vi "tvac_gui_v3.vi"() -> ()   [LabVIEW 2016]
uses:
  <vilib>/httpClient/LabVIEWHTTPClient.lvlib
  <vilib>/httpClient/ClientHandle.ctl
  msg7171_linux.llb/send single message.vi
  <vilib>/httpClient/POSTBuffer.vi
panel:
  in  "alarm":i32
  in  "NumberTCs":i32=10
  in  "Tab Control":enum32{"Page 1", "Page 2"}(tab)
  in  "Zone 1":T1 {"Ring" items=["Average", "Maximum", "Minimum", ""]}
  in  "Graphing Selection":u16(ring) items=["User Selection", "Graph All Thermocouples", "Clear Graph"]
  in  "Time Scale":u16(ring) items=["Minutes", "Hours", "Seconds"]
  out "Waveform Chart":waveform(dbl)[](graph)
  out "Thermocouples":T2(array[cluster])
  in  "exit":bool
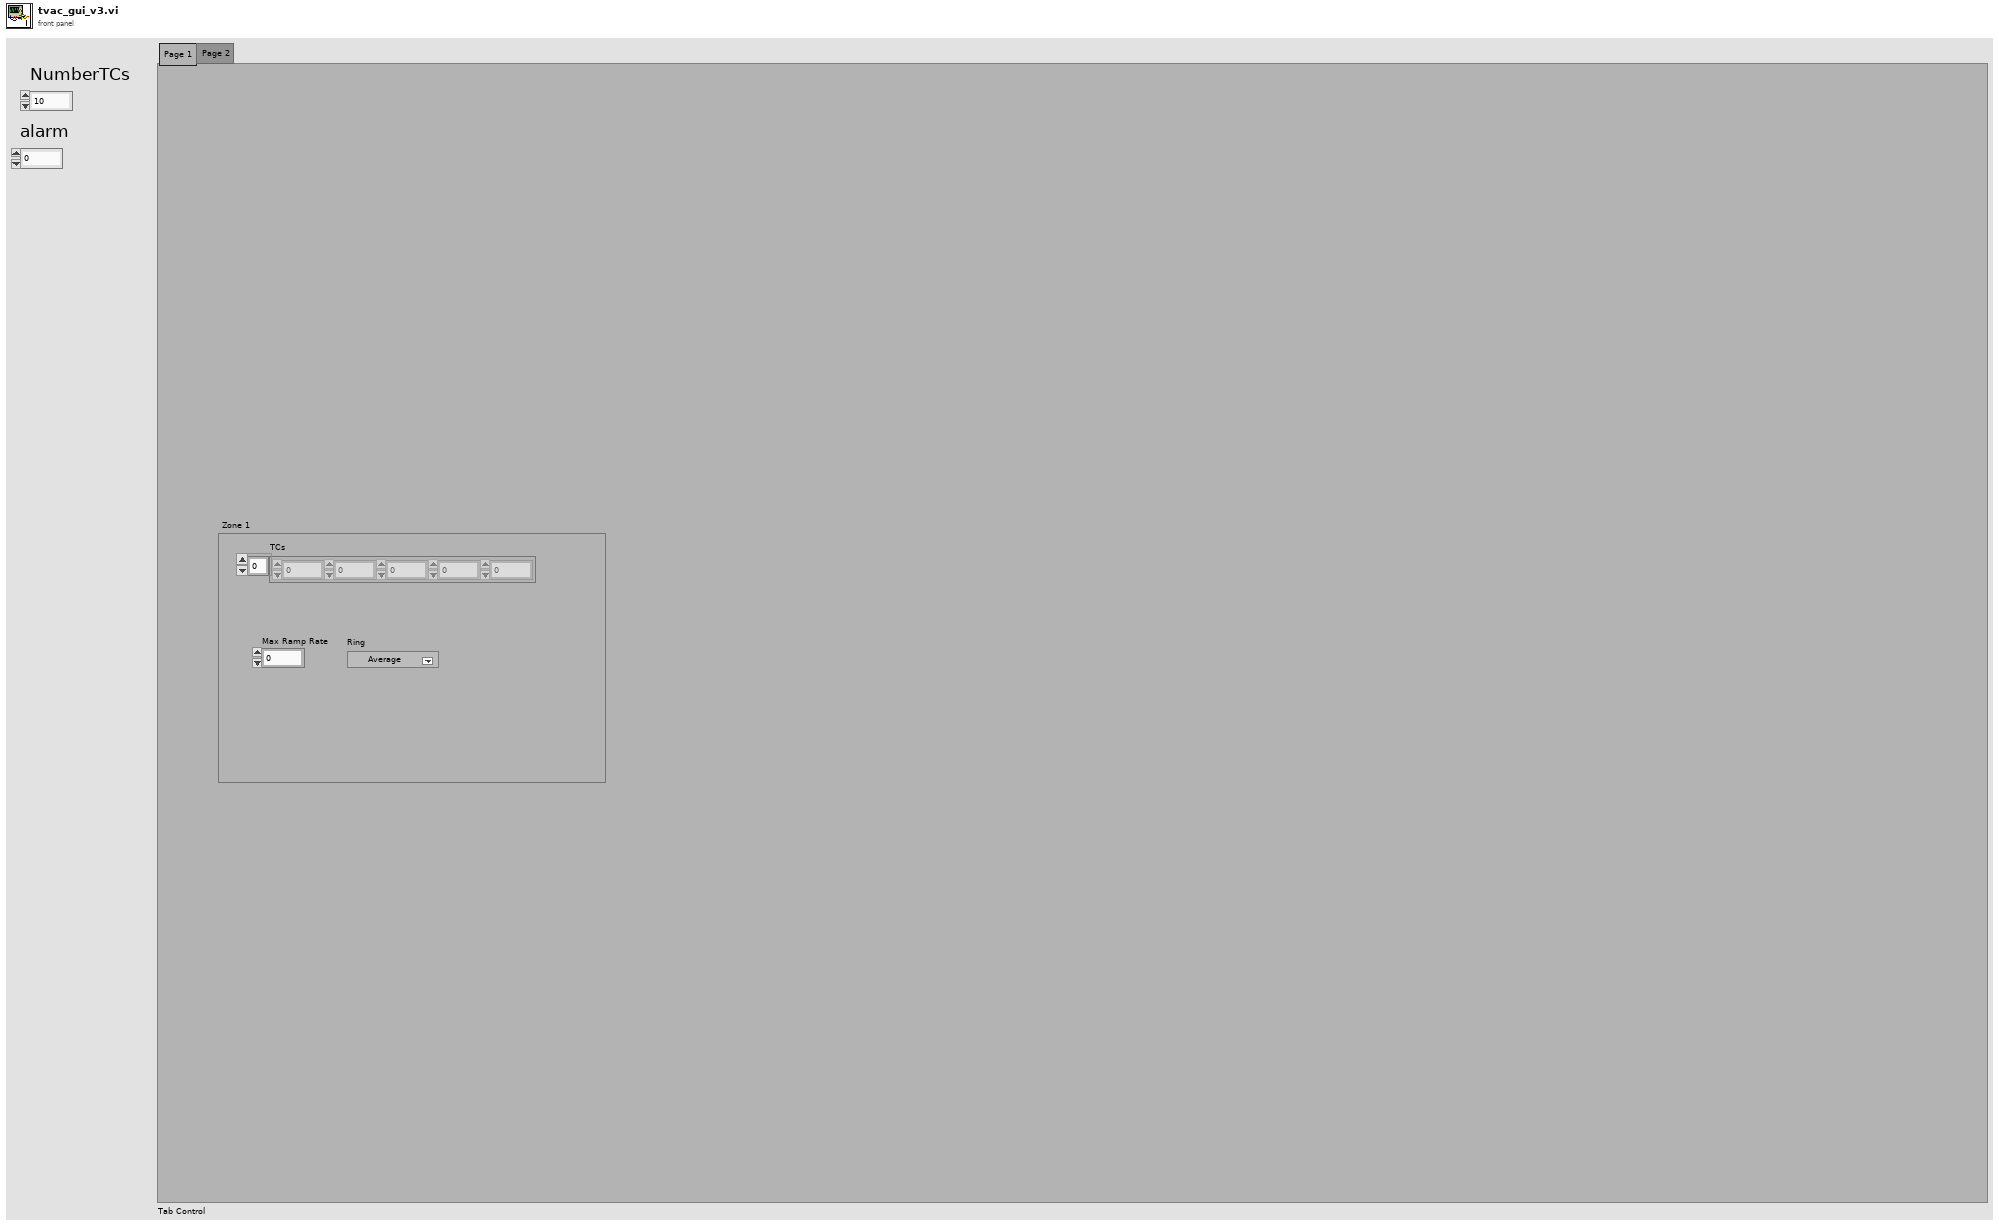
[diagram p1: front panel]
types:
  T1 = cluster{"Ring":u16, "Max Ramp Rate":dbl, "TCs":dbl[]}
  T2 = cluster{"TC Label":string, "Alarm Status":string, "Alarm Color":u32, "Temperature":string, "PlotColor":u32, "Graph On/Off":u32}[][]
  T3 = typedef "LabVIEWHTTPClient.lvlib/ClientHandle.ctl" = refnum<k1>
  T4 = cluster{"go":bool, "Http session":T3, "URL prefex":string}
  T5 = typedef "LVPoint32TypeDef.ctl" = cluster{"Horizontal":i32, "Vertical":i32}
  T6 = typedef "LVPositionTypeDef.ctl" = cluster{"Left":i32, "Top":i32}
  T7 = cluster{"TC Label":string, "Alarm Status":string, "Alarm Color":u32, "Temperature":string, "PlotColor":u32, "Graph On/Off":u32}
  T8 = typedef "LVRangeTypeDef.ctl" = cluster{"Minimum":dbl, "Maximum":dbl, "Increment":dbl, "Minor Increment":dbl, "Start":dbl}
  T9 = cluster{"time":string, "tcs":cluster{"thermocouple":i32, "time":i32, "temp":i32, "working":i32, "alarm":i32}[]}
  T10 = cluster{"thermocouple":i32, "time":i32, "temp":i32, "working":i32, "alarm":i32}[]
  T11 = cluster{"thermocouple":i32, "time":i32, "temp":i32, "working":i32, "alarm":i32}
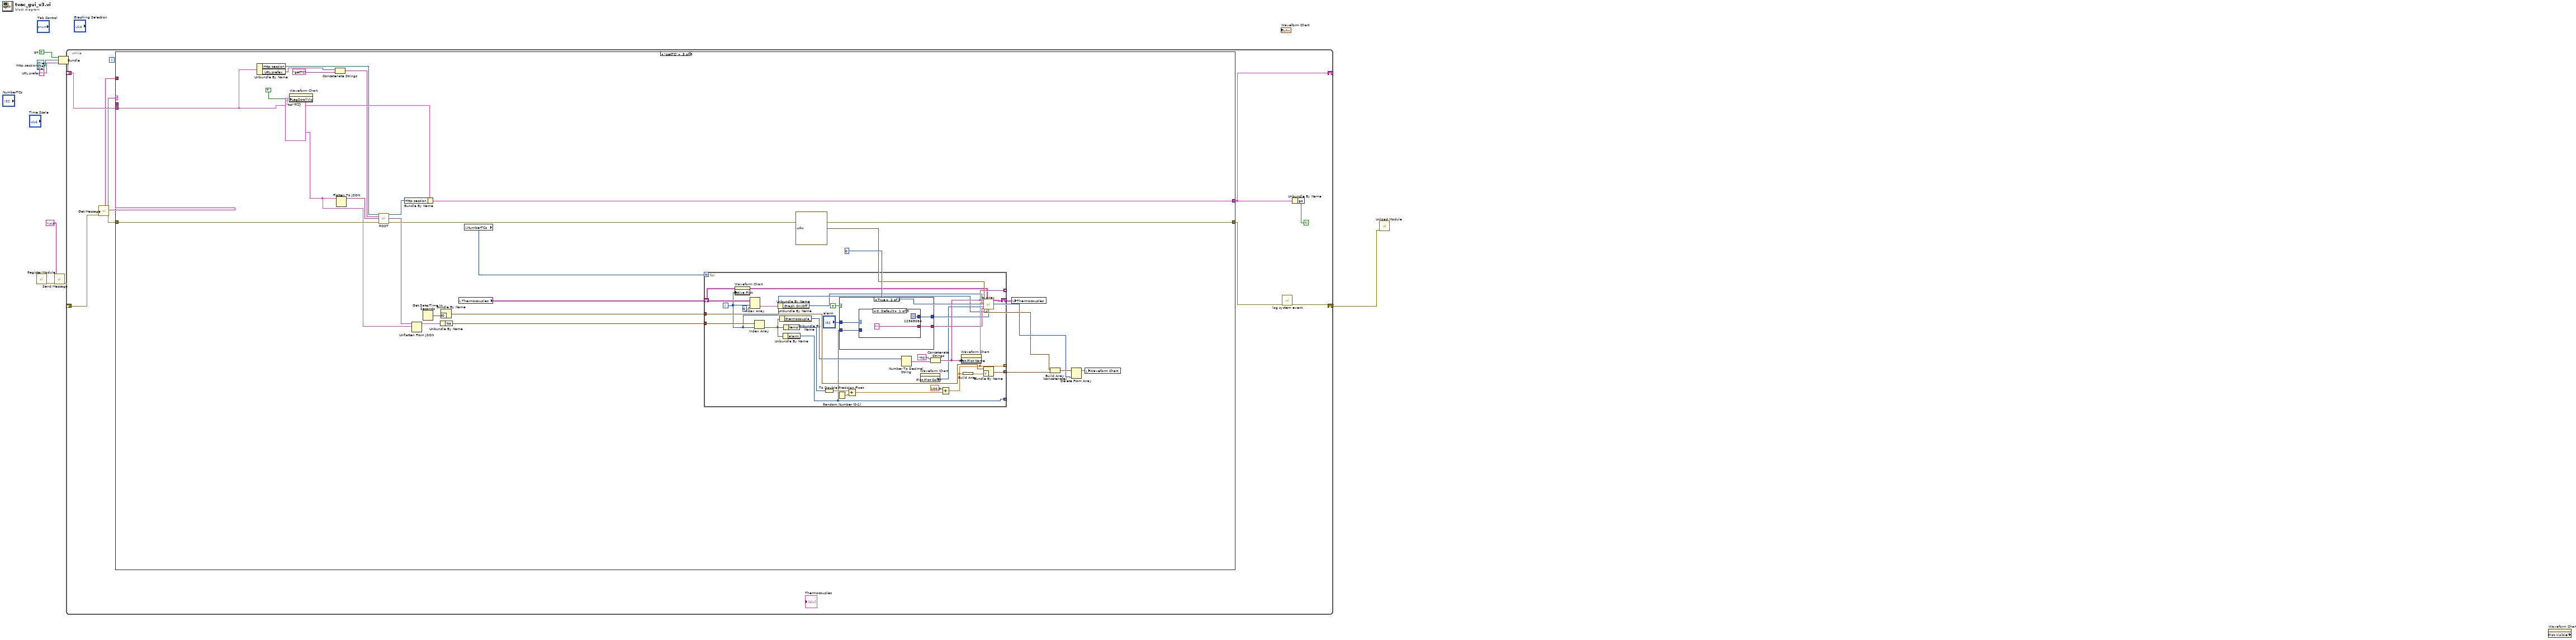
[diagram p0: block diagram]
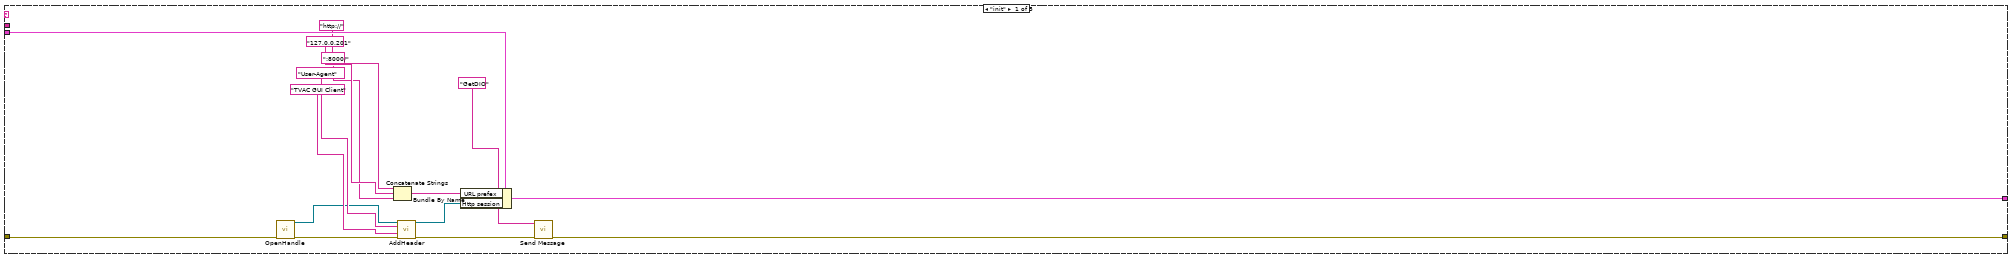
[diagram p2: hidden frame]
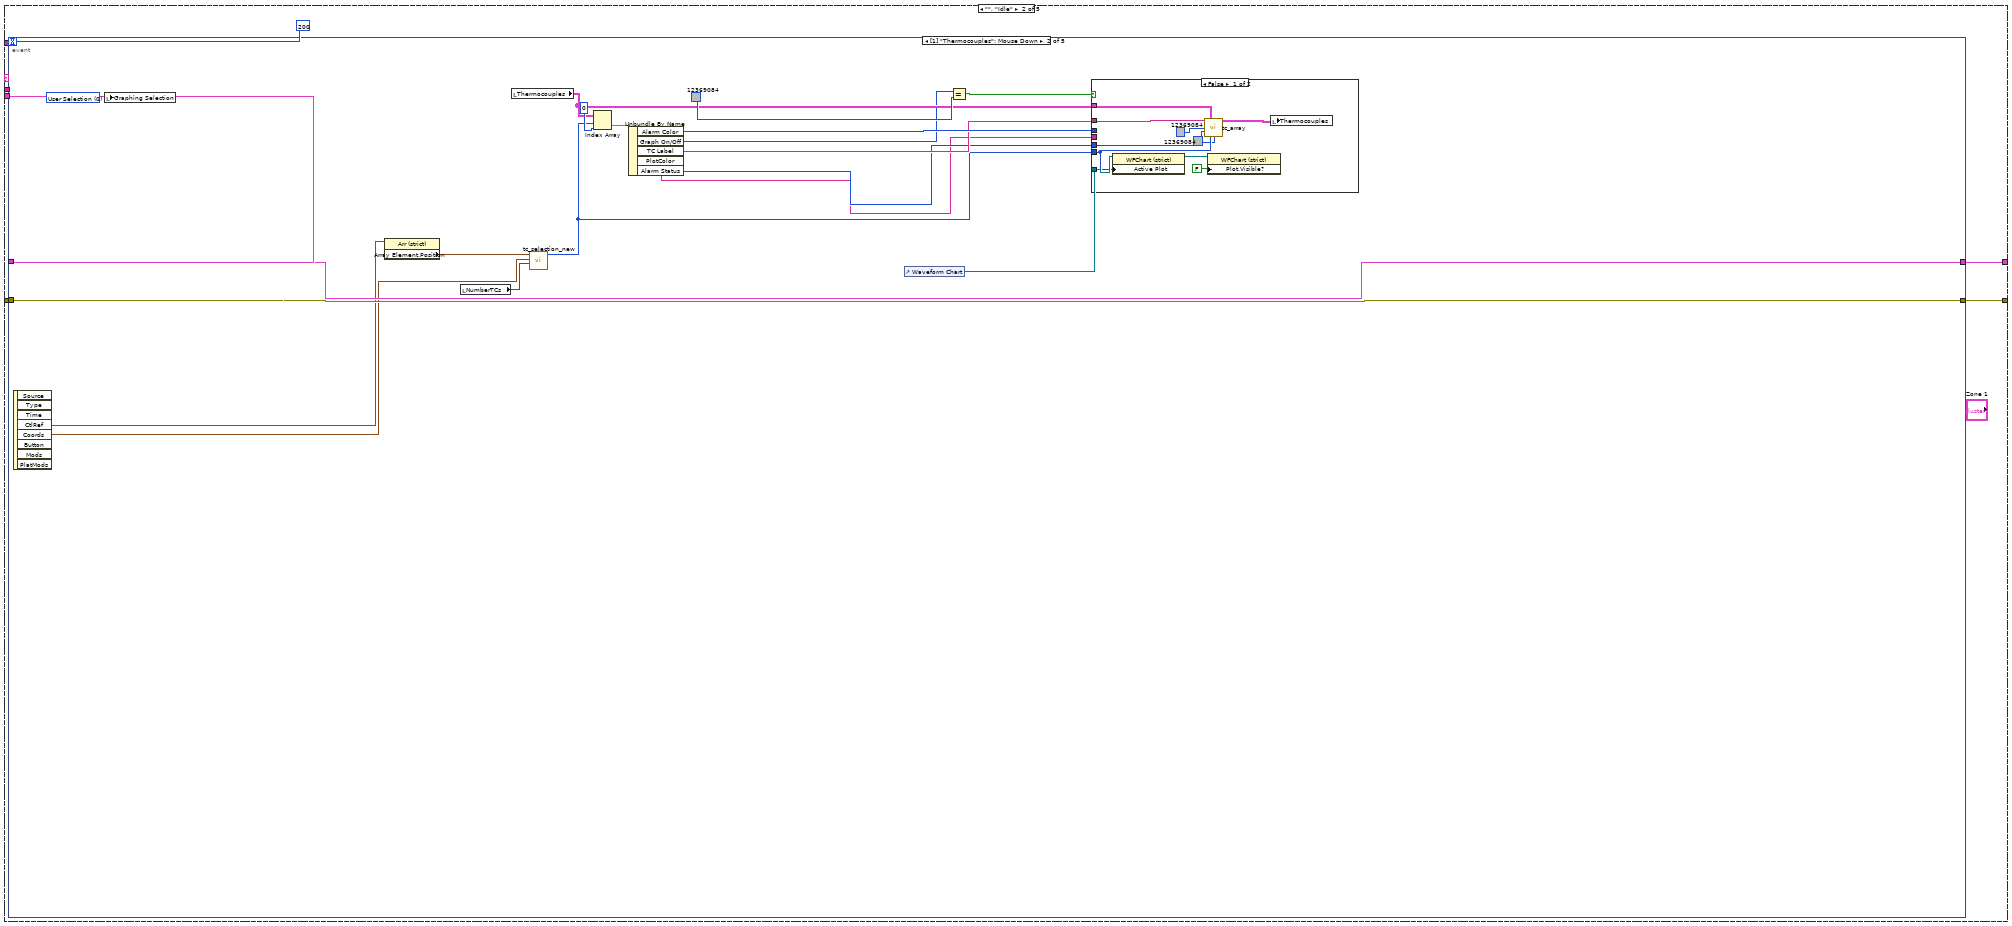
[diagram p3: hidden frame]
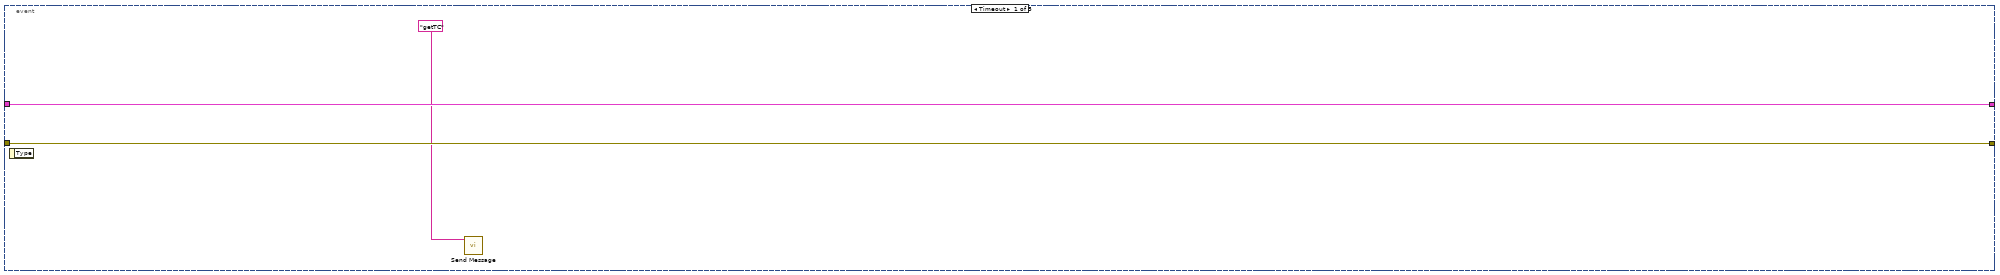
[diagram p4: hidden frame]
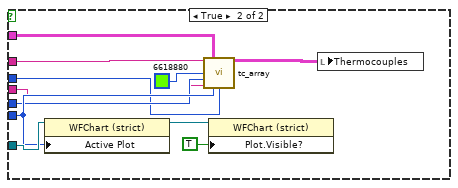
[diagram p5: hidden frame]
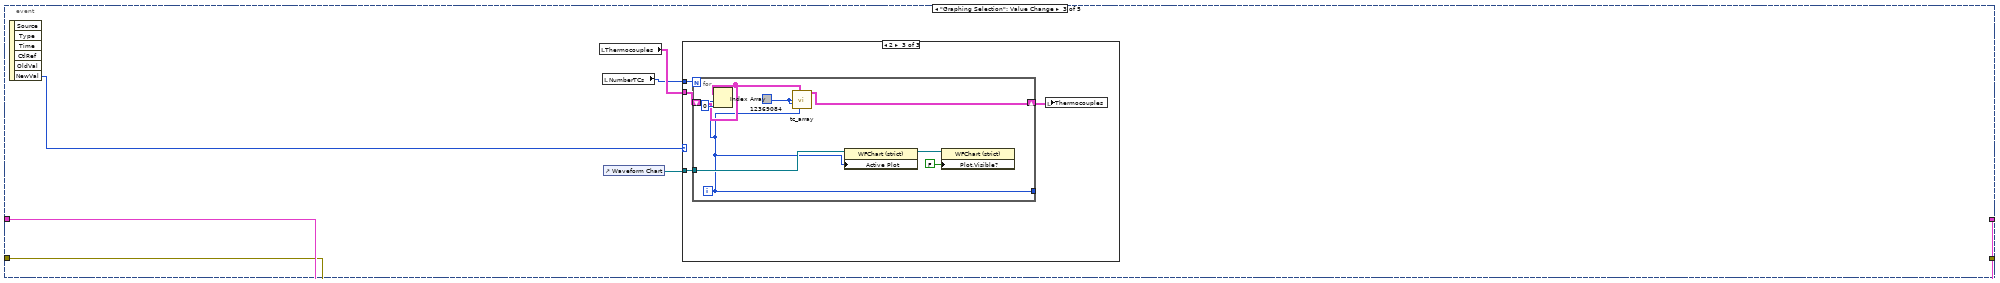
[diagram p6: hidden frame]
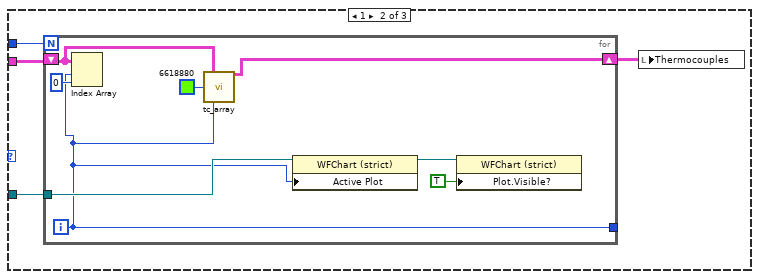
[diagram p8: hidden frame]
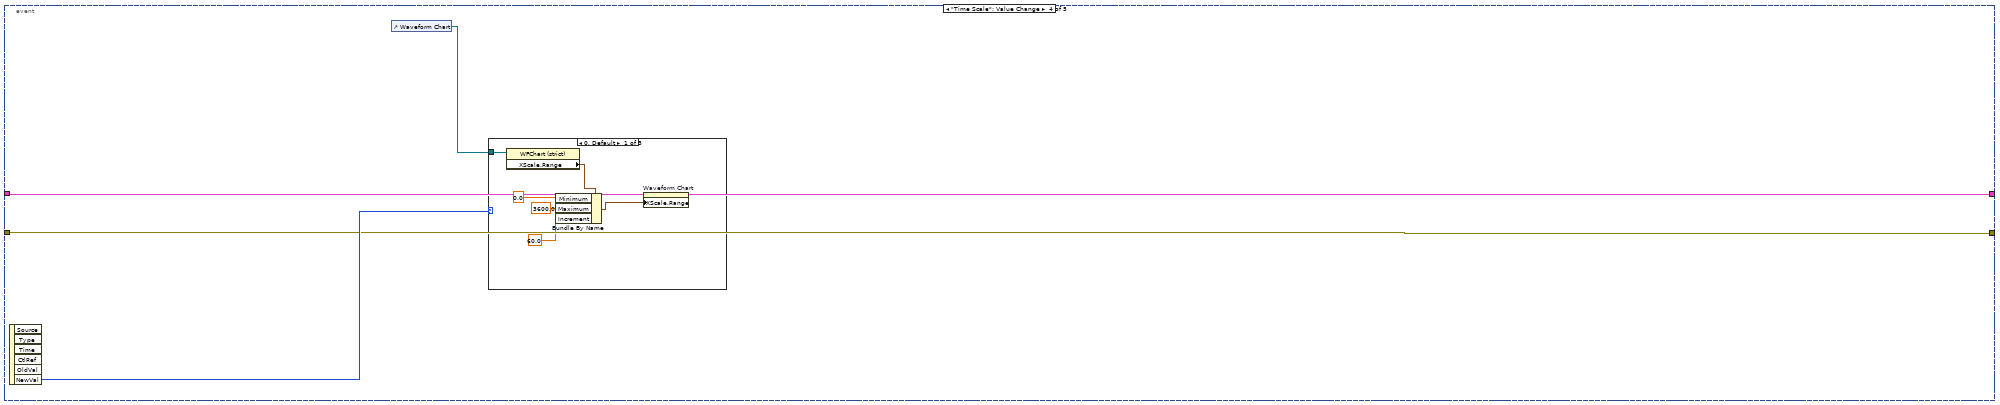
[diagram p9: hidden frame]
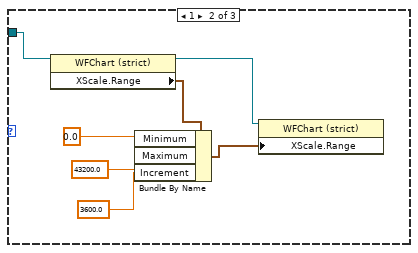
[diagram p10: hidden frame]
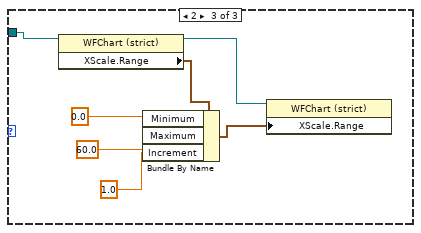
[diagram p11: hidden frame]
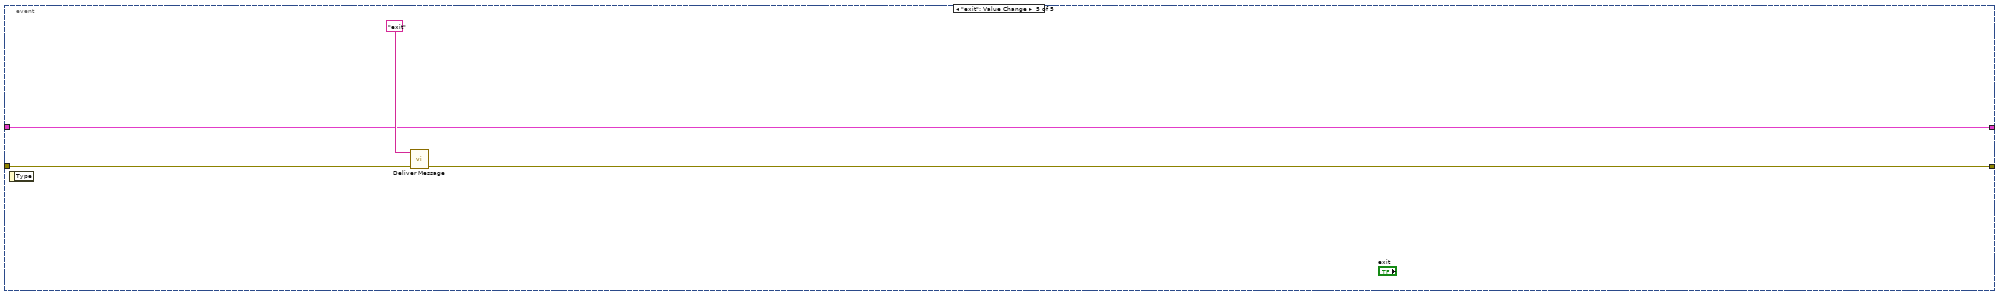
[diagram p12: hidden frame]
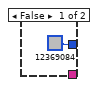
[diagram p13: hidden frame]
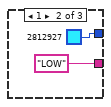
[diagram p14: hidden frame]
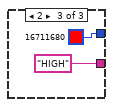
[diagram p15: hidden frame]
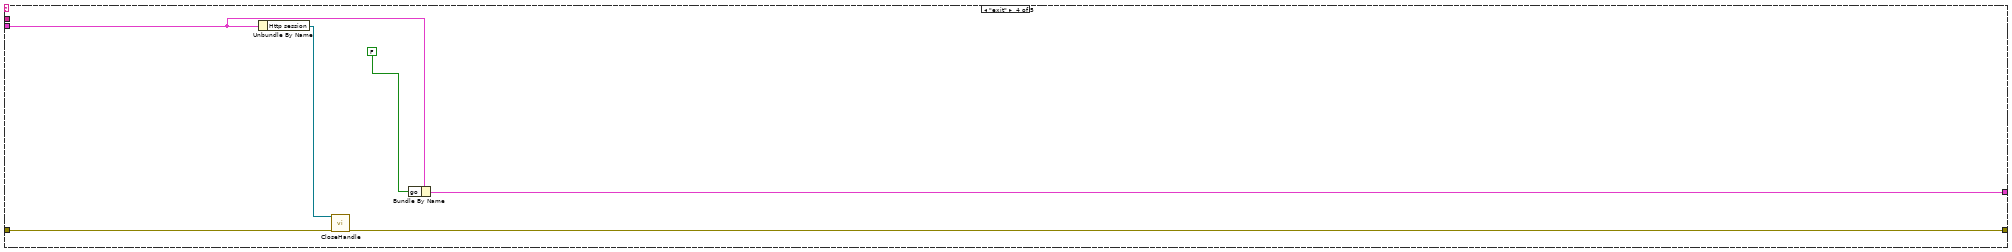
[diagram p16: hidden frame]
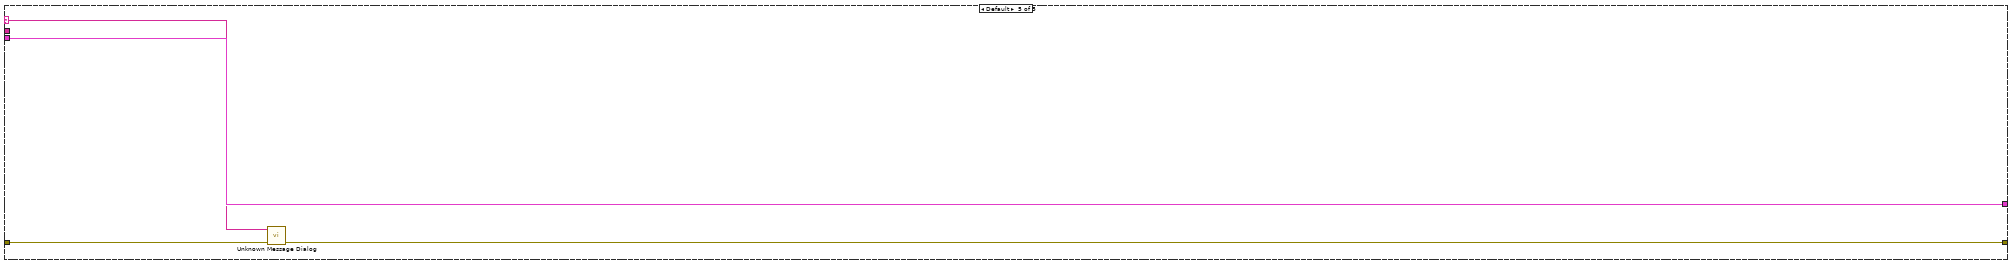
[diagram p17: hidden frame]
diagram:
  w4 = ""  # URL prefex
  w5 = T3 refnum  # Http session
  w6 = TRUE  # go
  n1 = call "Register Module.vi"() -> ("error out"=w2:errorcluster)  [unwired: 10 in, 1 out]
  n2 = call-poly "Send Message.vi"("error in (no error)"=w2, "event"="init") -> ("error out"=w1:errorcluster)  [unwired: 9 in]
  n3 = Bundle("go"=w6, "Http session"=w5, "URL prefex"=w4) -> (w8:T4)  [unwired: 1 in]
  n4 = while {
    shift-left: w8 -> [w15]
    shift-right: [w13] -> _
    shift-right: [w12] -> w7
    shift-left: w1 -> [w18]
    stop <- w9 continue-if-true
    n5 = call "Get Message.vi"("error in (no error)"=w18) -> ("error out"=w16:errorcluster, "event buffer"=w17:string, "event"=w14:string, "source"=w10:string)  [unwired: 7 in]
    n6 = case shown="\"getTC\"" w14 {
      selector: w14 -> [_ _ _ _ w210]
      tunnel: [w24 w35 w162 w208 w212] -> w13
      tunnel: w15 -> [w33 w34 w160 w203 w212]
      tunnel: w17 -> [_ _ _ _ _]
      tunnel: w16 -> [w28 w36 w164 w206 w211]
      tunnel: [w20 w38 w163 w205 w209] -> w11
      tunnel: w10 -> [_ _ _ _ _]
      frame "init" {
        n7 = call <vilib>:"OpenHandle.vi"("error in (no error)"=w28) -> ("client handle out"=w29:T3, "error out"=w32:errorcluster)  [unwired: 13 in]
        n8 = Concatenate Strings("http://" ("url"), "127.0.0.201" ("Address"), ":8000/" ("url")) -> (w23:string)
        n9 = call <vilib>:"AddHeader.vi"("client handle"=w29, "header"="User-Agent", "value"="TVAC GUI Client", "error in (no error)"=w32) -> ("client handle out"=w22:T3, "error out"=w21:errorcluster)  [unwired: 10 in]
        n10 = Bundle By Name(cluster=w33, "URL prefex"=w23, "Http session"=w22) -> (w24:T4)
        n11 = call-poly "Send Message.vi"("error in (no error)"=w21, "event"="GetDIO") -> ("error out"=w20:errorcluster)  [unwired: 9 in]
      }
      frame "", "Idle" {
        n12 = event shown="[1] \"Thermocouples\": Mouse Down" {
          selector: _ -> [_ _ _ _ _]
          dyn-events: _ -> [_ _ _ _ _]
          timeout: 200 ("milliseconds to wait") -> [_ _ _ _ _]
          tunnel: w36 -> [w40 w60 w86 w113 w139]
          tunnel: [w40 w60 w86 w113 w138] -> w38
          tunnel: [w41 w59 w87 w114 w136] -> w35
          tunnel: w34 -> [w41 w59 w87 w114 w136]
          event Timeout {
            n13 = event-data() -> ()  [unwired: 1 in, 1 out]
            n14 = call-poly "Send Message.vi"("event"="getTC") -> ()  [unwired: 10 in, 1 out]
          }
          event "Thermocouples": Mouse Down {
            w42 = u16 0 items=["User Selection", "Graph All Thermocouples", "Clear Graph"] ("Graphing Selection")
            n15 = event-data() -> ("CtlRef"=w56:refnum<vi>, "Coords"=w57:T5)  [unwired: 1 in, 6 out]
            n16 = local write "Graphing Selection"(w42) -> ()
            n17 = property class="Arr (strict)"(reference=w56) -> ("Array Element.Position"=w58:T6)  [unwired: 1 in, 2 out]
            n18 = local read "NumberTCs"() -> (w48:i32)
            n19 = local read "Thermocouples"() -> (w50:T2)
            n20 = call "tc_selection_new.vi"("Numeric 2"=w48, "Coords"=w57, "Position"=w58) -> ("Numeric"=w44:i32)  [unwired: 8 in]
            n21 = Index Array(array=w50, index (row)=w44, index (col)=0 ("disabled index (col)")) -> (element=w53:T7)
            n22 = Unbundle By Name(w53) -> ("Alarm Color"=w49:u32, "Graph On/Off"=w47:u32, "TC Label"=w46:string, "PlotColor"=w45:u32, "Alarm Status"=w43:string)
            n23 = control-ref of="Waveform Chart"() -> (w51:refnum<vi>)
            n24 = Equal?(x=w47, y=u32 12369084) -> (x = y?=w52:bool)
            n25 = case shown="False" w52 {
              tunnel: w44 -> [w62 w74]
              tunnel: w51 -> [w68 w79]
              tunnel: w50 -> [w64 w76]
              tunnel: w49 -> [_ w72]
              tunnel: w46 -> [w66 w78]
              tunnel: w45 -> [w63 w73]
              tunnel: w43 -> [_ w71]
              frame False {
                n26 = property on="Property Node" class="WFChart (strict)"(reference=w68, "Active Plot"=w62) -> (reference out=w69:refnum<vi>)  [unwired: 1 in, 1 out]
                n27 = call "tc_array.vi"("TC Label"=w66, "output array 2"=w64, "Graph ON/OFF"=u32 12369084, "Plot Color"=w63, "index (row)"=w62, "AlarmColor"=u32 12369084) -> ("output array"=w65:T2)  [unwired: 9 in]
                n28 = property class="WFChart (strict)"(reference=w69, "Plot.Visible?"=FALSE ("Plot.Visible")) -> ()  [unwired: 1 in, 2 out]
                n29 = local write "Thermocouples"(w65) -> ()
              }
              frame True {
                n30 = property class="WFChart (strict)"(reference=w79, "Active Plot"=w74) -> (reference out=w80:refnum<vi>)  [unwired: 1 in, 1 out]
                n31 = call "tc_array.vi"("TC Label"=w78, "output array 2"=w76, "Graph ON/OFF"=u32 6618880, "Plot Color"=w73, "Alarm String"=w71, "index (row)"=w74, "AlarmColor"=w72) -> ("output array"=w75:T2)  [unwired: 8 in]
                n32 = property class="WFChart (strict)"(reference=w80, "Plot.Visible?"=TRUE ("Plot.Visible")) -> ()  [unwired: 1 in, 2 out]
                n33 = local write "Thermocouples"(w75) -> ()
              }
            }
          }
          event "Graphing Selection": Value Change {
            n34 = event-data() -> ("NewVal"=w82:u16)  [unwired: 1 in, 5 out]
            n35 = local read "Thermocouples"() -> (w85:T2)
            n36 = local read "NumberTCs"() -> (w83:i32)
            n37 = control-ref of="Waveform Chart"() -> (w84:refnum<vi>)
            n38 = case shown="2" w82 {
              tunnel: w85 -> [_ w91 w102]
              tunnel: w84 -> [_ w90 w101]
              tunnel: w83 -> [_ w89 w103]
              frame 0, Default {
              }
              frame 1 {
                n39 = for {
                  N: w89 -> [_]
                  tunnel: w90 -> [w96]
                  tunnel: [w95] -> _
                  shift-right: [w93] -> w88
                  shift-left: w91 -> [w94]
                  i -> [w95]
                  n40 = Index Array(array=w94, index (row)=w95, index (col)=0 ("disabled index (col)")) -> ()  [unwired: 1 out]
                  n41 = call "tc_array.vi"("output array 2"=w94, "Graph ON/OFF"=u32 6618880, "index (row)"=w95) -> ("output array"=w93:T2)  [unwired: 12 in]
                  n42 = property class="WFChart (strict)"(reference=w96, "Active Plot"=w95) -> (reference out=w98:refnum<vi>)  [unwired: 1 in, 1 out]
                  n43 = property class="WFChart (strict)"(reference=w98, "Plot.Visible?"=TRUE ("Plot.Visible")) -> ()  [unwired: 1 in, 2 out]
                }
                n44 = local write "Thermocouples"(w88) -> ()
              }
              frame 2 {
                n45 = for {
                  N: w103 -> [_]
                  tunnel: w101 -> [w108]
                  tunnel: [w106] -> _
                  shift-right: [w104] -> w100
                  shift-left: w102 -> [w107]
                  i -> [w106]
                  w105 = u32 12369084
                  n46 = Index Array(array=w107, index (row)=w106, index (col)=0 ("disabled index (col)")) -> ()  [unwired: 1 out]
                  n47 = call "tc_array.vi"("output array 2"=w107, "Graph ON/OFF"=w105, "Plot Color"=w105, "index (row)"=w106) -> ("output array"=w104:T2)  [unwired: 11 in]
                  n48 = property class="WFChart (strict)"(reference=w108, "Active Plot"=w106) -> (reference out=w110:refnum<vi>)  [unwired: 1 in, 1 out]
                  n49 = property class="WFChart (strict)"(reference=w110, "Plot.Visible?"=FALSE ("Plot.Visible")) -> ()  [unwired: 1 in, 2 out]
                }
                n50 = local write "Thermocouples"(w100) -> ()
              }
            }
          }
          event "Time Scale": Value Change {
            n51 = event-data() -> ("NewVal"=w115:u16)  [unwired: 1 in, 5 out]
            n52 = control-ref of="Waveform Chart"() -> (w112:refnum<vi>)
            n53 = case shown="0, Default" w115 {
              tunnel: w112 -> [w119 w123 w130]
              frame 0, Default {
                n54 = property on="Property Node" class="WFChart (strict)"(reference=w119) -> ("XScale.Range"=w121:T8)  [unwired: 1 in, 2 out]
                n55 = Bundle By Name(cluster=w121, "Minimum"=0.0, "Maximum"=3600.0, "Increment"=60.0) -> (w120:T8)
                n56 = property on="Waveform Chart" class="WFChart (strict)"("XScale.Range"=w120) -> ()  [unwired: 2 in, 2 out]
              }
              frame 1 {
                n57 = property on="Property Node" class="WFChart (strict)"(reference=w123) -> (reference out=w122:refnum<vi>, "XScale.Range"=w128:T8)  [unwired: 1 in, 1 out]
                n58 = Bundle By Name(cluster=w128, "Minimum"=0.0, "Maximum"=43200.0, "Increment"=3600.0) -> (w124:T8)
                n59 = property on="Property Node" class="WFChart (strict)"(reference=w122, "XScale.Range"=w124) -> ()  [unwired: 1 in, 2 out]
              }
              frame 2 {
                n60 = property on="Property Node" class="WFChart (strict)"(reference=w130) -> (reference out=w129:refnum<vi>, "XScale.Range"=w135:T8)  [unwired: 1 in, 1 out]
                n61 = Bundle By Name(cluster=w135, "Minimum"=0.0, "Maximum"=60.0, "Increment"=1.0) -> (w131:T8)
                n62 = property on="Property Node" class="WFChart (strict)"(reference=w129, "XScale.Range"=w131) -> ()  [unwired: 1 in, 2 out]
              }
            }
          }
          event "exit": Value Change {
            n63 = event-data() -> ()  [unwired: 1 in, 1 out]
            n64 = call "Deliver Message.vi"("error in (no error)"=w139, "event"="exit") -> ("error out"=w138:errorcluster)  [unwired: 9 in]
          }
        }
      }
      frame "getTC" {
        w153 = T9 {"time"="", "tcs"=[]}
        n65 = Unbundle By Name(w160) -> ("Http session"=w159:T3, "URL prefex"=w157:string)
        n66 = property on="Waveform Chart" class="WFChart (strict)"("LegScrollVis"=TRUE ("Legend:Scrollbar Visible")) -> ()  [unwired: 2 in, 2 out]
        n67 = Concatenate Strings(w157, "getTC" ("url")) -> (w158:string)
        n68 = Flatten To JSON(anything=w153) -> (JSON string=w155:string)  [unwired: 2 in, 1 out]
        n69 = call-poly <vilib>:"POST.vi"("client handle"=w159, "url"=w158, "buffer"=w155, "error in (no error)"=w164) -> ("client handle out"=w161:T3, "body"=w154:string, "error out"=w163:errorcluster)  [unwired: 8 in, 1 out]
        n70 = Bundle By Name(cluster=w160, "Http session"=w161) -> (w162:T4)
        n71 = Unflatten From JSON(JSON string=w154, type and defaults=w153) -> (value=w152:T9)  [unwired: 5 in, 1 out]
        n72 = Get Date/Time In Seconds() -> (seconds since 1Jan1904=w148:timestamp)
        n73 = Unbundle By Name(w152) -> ("tcs"=w151:T10)
        n74 = Bundle By Name("t0"=w148) -> (w147:waveform(dbl))  [unwired: 1 in]
        n75 = local read "Thermocouples"() -> (w143:T2)
        n76 = local read "NumberTCs"() -> (w140:i32)
        n77 = for {
          N: w140 -> [_]
          tunnel: w151 -> [w191]
          tunnel: w147 -> [w189]
          tunnel: [w190] -> w146 mode=indexing
          tunnel: [w172] -> _ mode=indexing
          tunnel: [w171] -> _ mode=indexing
          tunnel: [w174] -> _ mode=indexing
          shift-right: [w173] -> w144
          shift-left: w143 -> [w170]
          i -> [w167]
          n78 = property on="Waveform Chart" class="WFChart (strict)"("Active Plot"=w167) -> ()  [unwired: 2 in, 2 out]
          n79 = Index Array(array=w170, index (row)=w167, index (col)=0 ("disabled index (col)")) -> (element=w177:T7)
          n80 = Index Array(array=w191, index=w167) -> (element=w181:T11)
          n81 = Unbundle By Name(w177) -> ("Graph On/Off"=w165:u32)
          n82 = Unbundle By Name(w181) -> ("thermocouple"=w187:i32)
          n83 = Unbundle By Name(w181) -> ("alarm"=w174:i32)
          n84 = Unbundle By Name(w181) -> ("temp"=w185:i32)
          n85 = To Double Precision Float(number=w185) -> (double precision float=w182:dbl)
          n86 = Random Number (0-1)() -> (number: 0 to 1=w183:dbl)
          n87 = case shown="True" TRUE {
            tunnel: [_ w196] -> w169
            tunnel: "alarm" -> [_ w195]
            tunnel: w174 -> [_ w194]
            tunnel: [u32 12369084 w193] -> w168
            frame False {
            }
            frame True {
              n88 = case shown="0, Default" w195 {
                tunnel: ["" "LOW" "HIGH"] -> w196
                tunnel: w194 -> [_ _ _]
                tunnel: [u32 12369084 u32 2812927 u32 16711680] -> w193
                frame 0, Default {
                }
                frame 1 {
                }
                frame 2 {
                }
              }
            }
          }
          n89 = Add(x=w182, y=w183) -> (x+y=w179:dbl)
          n90 = Number To Decimal String(number=w187) -> (decimal integer string=w188:string)  [unwired: 1 in]
          n91 = property on="Waveform Chart" class="WFChart (strict)"() -> ("Plot.Plot Color"=w166:u32)  [unwired: 2 in, 2 out]
          n92 = Concatenate Strings("TC " ("string"), w188) -> (w171:string)
          n93 = Add(x=100.0, y=w179) -> (x+y=w172:dbl)
          n94 = property on="Waveform Chart" class="WFChart (strict)"("Plot.Plot Name"=w171) -> ()  [unwired: 2 in, 2 out]
          n95 = Build Array(w172) -> (w184:dbl[])
          n96 = call "tc_array.vi"("TC Label"=w171, "output array 2"=w170, "Temperature"=w172, "Graph ON/OFF"=w165, "Plot Color"=w166, "Alarm String"=w169, "index (row)"=w167, "AlarmColor"=w168) -> ("output array"=w173:T2)  [unwired: 7 in]
          n97 = Bundle By Name(cluster=w189, "Y"=w184) -> (w190:waveform(dbl))
        }
        n98 = local write "Thermocouples"(w144) -> ()
        n99 = Build Array (concatenate)(waveform(dbl) {"t0"=timestamp(0 s since 1904-01-01), "dt"=1.0, "Y"=[]} ("element"), w146) -> (w150:waveform(dbl)[])
        n100 = Delete From Array(array=w150, index=0) -> (array with subset deleted=w141:waveform(dbl)[])  [unwired: 1 in, 1 out]
        n101 = local write "Waveform Chart"(w141) -> ()
      }
      frame "exit" {
        n102 = Unbundle By Name(w203) -> ("Http session"=w204:T3)
        n103 = call <vilib>:"CloseHandle.vi"("client handle"=w204, "error in (no error)"=w206) -> ("error out"=w205:errorcluster)  [unwired: 13 in]
        n104 = Bundle By Name(cluster=w203, "go"=FALSE ("Bundle Element")) -> (w208:T4)
      }
      frame Default {
        n105 = call "Unknown Message Dialog.vi"("error in (no error)"=w211, "event name"=w210) -> ("error out"=w209:errorcluster)  [unwired: 9 in]
      }
    }
    n106 = call "log system event.vi"("error in (no error)"=w11) -> ("error out"=w12:errorcluster)  [unwired: 9 in, 1 out]
    n107 = Unbundle By Name(w13) -> ("go"=w9:bool)
  }
  n108 = call "Unload Module.vi"("error in (no error)"=w7) -> ()  [unwired: 10 in, 1 out]
  n109 = property on="Waveform Chart" class="WFChart (strict)" props=["Plot", "Visible?"]() -> ()  [unwired: 2 in, 3 out]
